vi "Configure Output.vi"(0 "VISA resource name":refnum<visa-resource-name>, 1 "Unit Address (1)":u8=1 min=1 max=254, 7 "Safe Output (0)":sgl min=-100 max=100 format="%.2g", 11 "error in (no error)":errorcluster, 12 "Manual Output (None:Track)":u16(ring) items=["None : TracK", "Step : Step", "Last : LastMOP"]) -> (4 "VISA resource name out":refnum<visa-resource-name>, 15 "error out":errorcluster)   [LabVIEW 2010, in "Eurotherm 32xx Series.lvlib"]
doc: "This VI sets Output Parameters."
uses:
  <instrlib>/Eurotherm 32xx Series/Eurotherm 32xx Series.lvlib
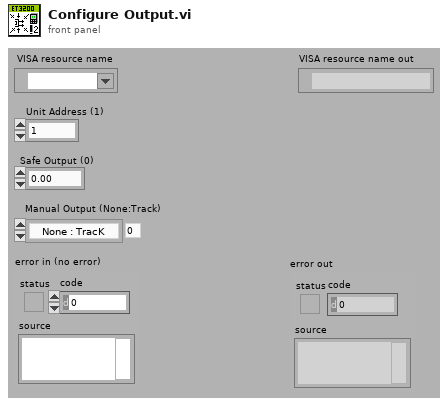
[diagram p1: front panel]
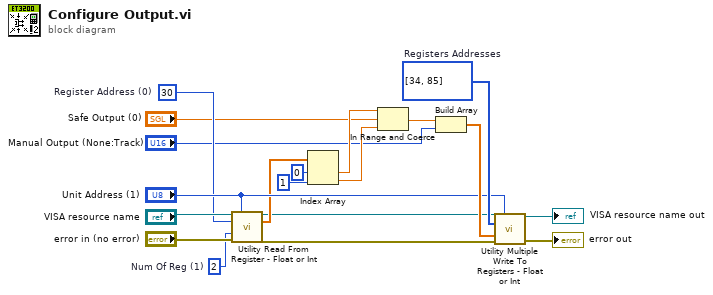
[diagram p0: block diagram]
diagram:
  w11 = u16 30  # Register Address (0)
  w12 = u16 2  # Num Of Reg (1)
  w16 = u16[] [34, 85]  # Registers Addresses
  n1 = call <instrlib>:"Utility Read From Register - Float or Int.vi"("VISA resource name"="VISA resource name", "Unit Address (1)"="Unit Address (1)", "Register Address (0)"=w11, "Num Of Reg (1)"=w12, "error in (no error)"="error in (no error)") -> ("VISA resource name out"=w4:refnum<visa-resource-name>, "Data"=w10:sgl[], "error out"=w3:errorcluster)  [unwired: 8 in]
  n2 = Index Array(array=w10, index #1=0 ("index"), index #2=1 ("index")) -> (element #1=w7:sgl, element #2=w6:sgl)
  n3 = In Range and Coerce(upper limit=w7, x="Safe Output (0)", lower limit=w6) -> (coerced(x)=w5:sgl)  [unwired: 1 out]
  n4 = Build Array(w5, "Manual Output (None:Track)") -> (w17:sgl[])
  n5 = call <instrlib>:"Utility Multiple Write To Registers - Float or Int.vi"("VISA resource name"=w4, "Unit Address (1)"="Unit Address (1)", "Registers Addresses (0)"=w16, "Data (0)"=w17, "error in (no error)"=w3) -> ("VISA resource name out"=→"VISA resource name out":refnum<visa-resource-name>, "error out"=→"error out":errorcluster)  [unwired: 9 in]
